vi "AprilTag position on field 2025.vi"(10 "AprilTag Number":i32=68) -> (2 "Target height to center (in)":dbl)   [LabVIEW 2025]
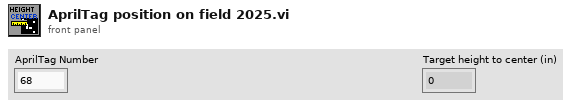
[diagram p1: front panel]
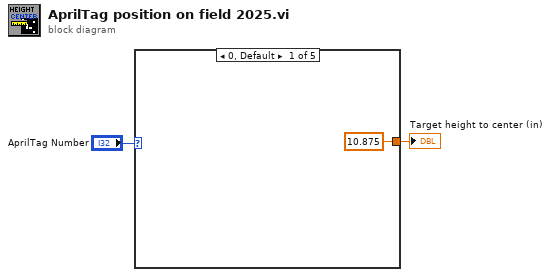
[diagram p0: block diagram]
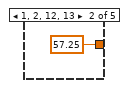
[diagram p2: hidden frame]
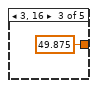
[diagram p3: hidden frame]
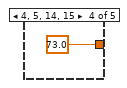
[diagram p4: hidden frame]
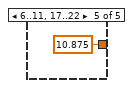
[diagram p5: hidden frame]
diagram:
  n1 = case shown="0, Default" "AprilTag Number" {
    tunnel: [10.875 57.25 49.875 73.0 10.875] -> w1
    frame 0, Default {
    }
    frame 1, 2, 12, 13 {
    }
    frame 3, 16 {
    }
    frame 4, 5, 14, 15 {
    }
    frame 6..11, 17..22 {
    }
  }
  "Target height to center (in)" <- w1
